vi "LV diagram otherobjs.vi"(11 "reference":refnum<vi>) -> (3 "String":string)   [LabVIEW 2012]
panel:
  out "Array":string[](array[string])
  out "unkn":cluster{i32, "UID":i32}[](array[cluster])
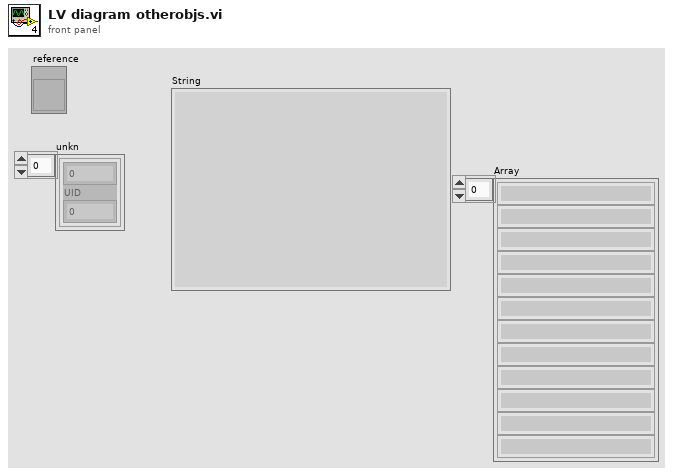
[diagram p1: front panel]
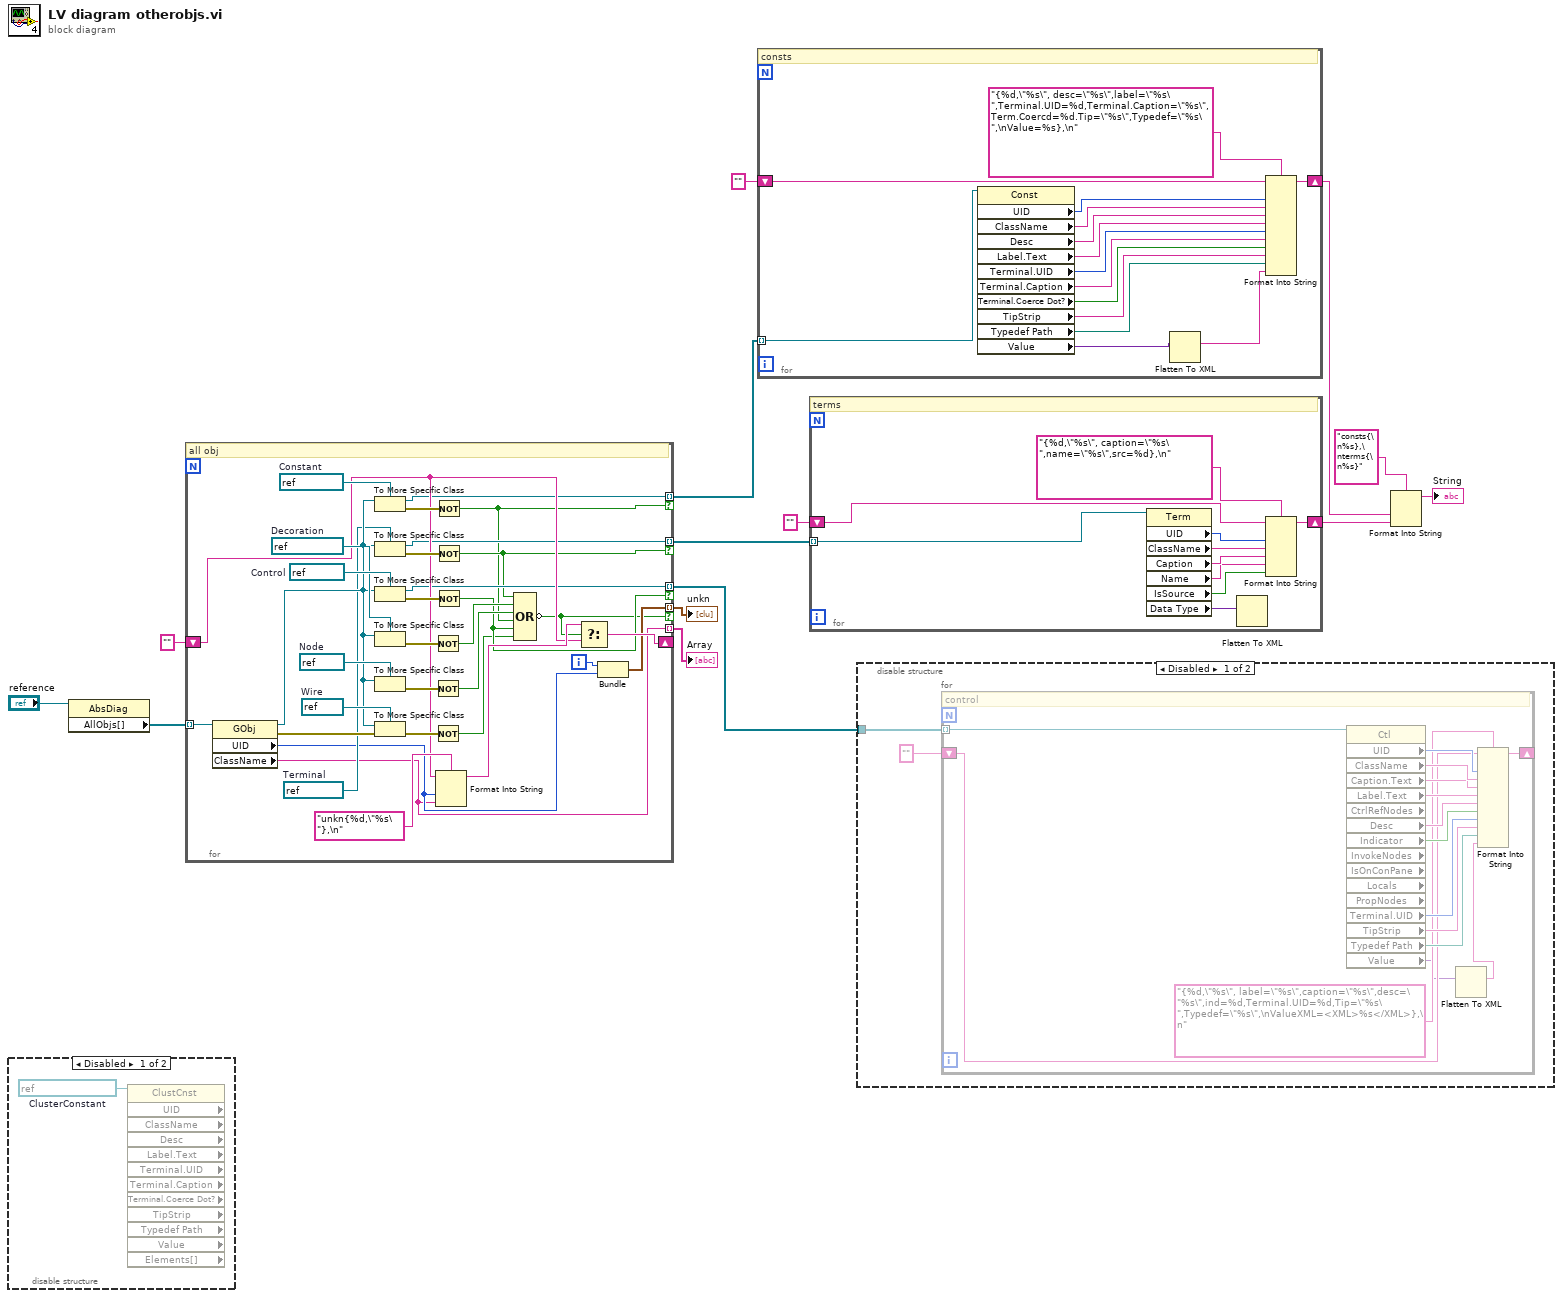
[diagram p0: block diagram]
diagram:
  n1 = disable-structure shown="Disabled" {
    frame Disabled {
      w15 = refnum<vi> refnum  # ClusterConstant
      n2 = property class="ClustCnst" props=["UID", "ClassName", "Desc", "Label", "Text", "Terminal", "UID", "Terminal", "Caption", "Terminal", "Coerce Dot?", "TipStrip", "Typedef Path", "Value", "Elements[]"](reference=w15) -> ()  [unwired: 1 in, 13 out]
    }
    frame Enabled {
    }
  }
  n3 = property class="AbsDiag"(reference="reference") -> ("AllObjs[]"=w13:refnum<vi>[])  [unwired: 1 in, 2 out]
  n4 = for {
    tunnel: [w26] -> w10 mode=indexing if=w20
    shift-right: [w30] -> _
    shift-left: "" -> [w31]
    tunnel: w13 -> [w34] mode=indexing
    tunnel: [w27] -> w11 mode=indexing if=w17
    tunnel: [w25] -> w9 mode=indexing if=w19
    tunnel: [w24] -> w8 mode=indexing if=w23
    tunnel: [w16] -> w6 mode=indexing
    i -> [w28]
    w36 = refnum<vi> refnum  # Terminal
    w42 = refnum<vi> refnum  # Node
    w43 = refnum<vi> refnum  # Decoration
    w44 = refnum<vi> refnum  # Control
    w45 = refnum<vi> refnum  # Constant
    w48 = refnum<vi> refnum  # Wire
    # "all obj"
    n5 = property class="GObj"(reference=w34) -> (reference out=w37:refnum<vi>, error out=w46:errorcluster, "UID"=w29:i32, "ClassName"=w16:string)  [unwired: 1 in]
    n6 = To More Specific Class(target class=w45, reference=w37) -> (specific class reference=w26:refnum<vi>, error out=w41:errorcluster)  [unwired: 1 in]
    n7 = To More Specific Class(target class=w36, reference=w37) -> (specific class reference=w24:refnum<vi>, error out=w35:errorcluster)  [unwired: 1 in]
    n8 = To More Specific Class(target class=w44, reference=w37) -> (specific class reference=w25:refnum<vi>, error out=w40:errorcluster)  [unwired: 1 in]
    n9 = To More Specific Class(target class=w43, reference=w37) -> (error out=w39:errorcluster)  [unwired: 1 in, 1 out]
    n10 = To More Specific Class(target class=w42, reference=w37) -> (error out=w38:errorcluster)  [unwired: 1 in, 1 out]
    n11 = To More Specific Class(target class=w48, reference=w37, error in=w46) -> (error out=w47:errorcluster)  [unwired: 1 out]
    n12 = Not(x=w39) -> (.not. x?=w22:bool)
    n13 = Not(x=w38) -> (.not. x?=w21:bool)
    n14 = Not(x=w47) -> (.not. x?=w18:bool)
    n15 = Not(x=w41) -> (.not. x?=w20:bool)
    n16 = Not(x=w35) -> (.not. x?=w23:bool)
    n17 = Not(x=w40) -> (.not. x?=w19:bool)
    n18 = Format Into String(format string="unkn{%d,\"%s\"},\n", initial string=w31, w29, w16) -> (resulting string=w32:string)  [unwired: 1 in, 1 out]
    n19 = Compound Arithmetic op=OR(w23, w22, w21, w20, w19, w18) -> (invert w17:bool)
    n20 = Select(t=w32, s=w17, f=w31) -> (s? t:f=w30:string)
    n21 = Bundle(w28, "UID"=w29) -> (w27:cluster{i32, "UID":i32})  [unwired: 1 in]
  }
  "unkn" <- w11
  "Array" <- w6
  n22 = for {
    tunnel: w10 -> [w63] mode=indexing
    shift-right: [w52] -> w4
    shift-left: "" -> [w53]
    # "consts"
    n23 = property class="Const"(reference=w63) -> ("UID"=w62:i32, "ClassName"=w61:string, "Desc"=w60:string, "Label.Text"=w59:string, "Terminal.UID"=w58:i32, "Terminal.Caption"=w57:string, "Terminal.Coerce Dot?"=w56:bool, "TipStrip"=w55:string, "Typedef Path"=w54:path, "Value"=w50:variant)  [unwired: 1 in, 2 out]
    n24 = Flatten To XML(anything=w50) -> (xml string=w49:string)
    n25 = Format Into String(format string="{%d,\"%s\", desc=\"%s\",label=\"%s\",Terminal.UID=%d,Terminal.Caption=\"%s\", Term.Coercd=%d.Tip=\"%s\",Typedef=\"%s\",\nValue=%s},\n", initial string=w53, w62, w61, w60, w59, w58, w57, w56, w55, w54, w49) -> (resulting string=w52:string)  [unwired: 1 in, 1 out]
  }
  n26 = for {
    tunnel: w8 -> [w73] mode=indexing
    shift-right: [w67] -> w3
    shift-left: "" -> [w66]
    # "terms"
    n27 = property class="Term"(reference=w73) -> ("UID"=w72:i32, "ClassName"=w71:string, "Caption"=w70:string, "Name"=w65:string, "IsSource"=w69:bool, "Data Type"=w64:variant)  [unwired: 1 in, 2 out]
    n28 = Flatten To XML(anything=w64) -> ()  [unwired: 1 out]
    n29 = Format Into String(format string="{%d,\"%s\", caption=\"%s\",name=\"%s\",src=%d},\n", initial string=w66, w72, w71, w70, w65, w69) -> (resulting string=w67:string)  [unwired: 1 in, 1 out]
  }
  n30 = disable-structure shown="Disabled" {
    disable-tunnel: w9 -> [w75 _]
    frame Disabled {
      n31 = for {
        tunnel: w75 -> [w90] mode=indexing
        shift-right: [w80] -> _
        shift-left: "" -> [w79]
        # "control"
        n32 = property class="Ctl" props=["UID", "ClassName", "Caption", "Text", "Label", "Text", "CtrlRefNodes", "Desc", "Indicator", "InvokeNodes", "IsOnConPane", "Locals", "PropNodes", "Terminal", "UID", "TipStrip", "Typedef Path", "Value"](reference=w90) -> ("UID"=w89:i32, "ClassName"=w88:string, "Caption.Text"=w87:string, "Label.Text"=w86:string, "Desc"=w85:string, "Indicator"=w84:bool, "Terminal.UID"=w83:i32, "TipStrip"=w82:string, "Typedef Path"=w81:path, "Value"=w77:variant)  [unwired: 1 in, 7 out]
        n33 = Flatten To XML(anything=w77) -> (xml string=w76:string)
        n34 = Format Into String(format string="{%d,\"%s\", label=\"%s\",caption=\"%s\",desc=\"%s\",ind=%d,Terminal.UID=%d,Tip=\"%s\",Typedef=\"%s\",\nValueXML=<XML>%s</XML>},\n", initial string=w79, w89, w88, w87, w86, w85, w84, w83, w82, w81, w76) -> (resulting string=w80:string)  [unwired: 1 in, 1 out]
      }
    }
    frame Enabled {
    }
  }
  n35 = Format Into String(format string="consts{\n%s},\nterms{\n%s}", w4, w3) -> (resulting string=→"String":string)  [unwired: 2 in, 1 out]
